vi "3D_plot.vi"(0 "Object Refnum In":refnum<vi>, 5 "error in (no error)":errorcluster, 7 "X":u16, 9 "Y":u16, 11 "Z":u16) -> (4 "3D Picture Control":refnum<vi>(3d-picture))   [LabVIEW 2012]
uses:
  <vilib>/Utility/miscctls.llb/LV3DPointTypeDef.ctl
  <vilib>/picture/3D Picture Control/NI_3D Picture Control.lvlib
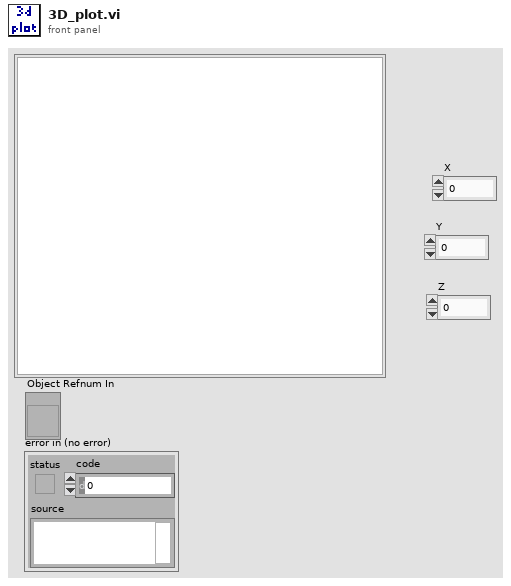
[diagram p1: front panel]
types:
  T1 = typedef "LV3DPointTypeDef.ctl" = cluster{"X":sgl, "Y":sgl, "Z":sgl}
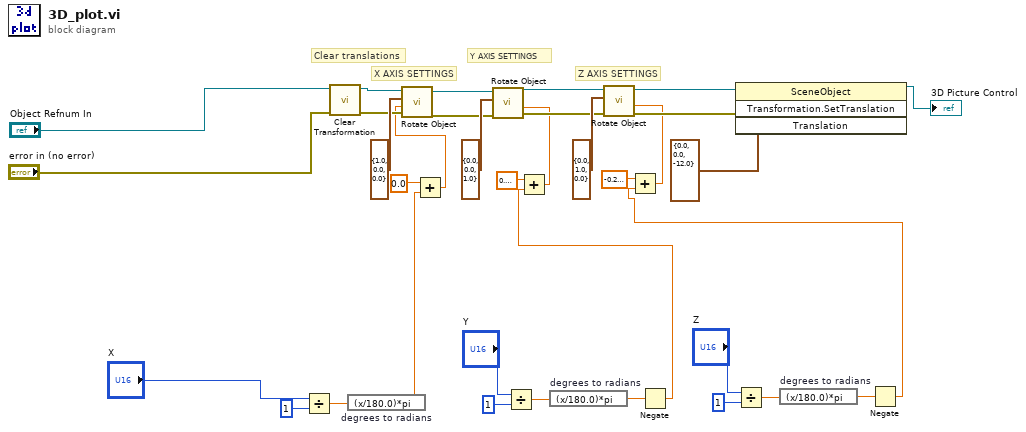
[diagram p0: block diagram]
diagram:
  # "Z AXIS SETTINGS"
  # "Y AXIS SETTINGS"
  # "Clear translations"
  # "X AXIS SETTINGS"
  n1 = Divide(x="X", y=1) -> (x/y=w15:dbl)
  n2 = call <vilib>:"Clear Transformation.vi"("error in (no error)"="error in (no error)", "Object Refnum In"="Object Refnum In") -> ("error out"=w24:errorcluster, "Object Refnum Out"=w34:refnum<vi>)  [unwired: 8 out]
  n3 = expression code="(x/180.0)*pi" "degrees to radians"(w15) -> (w14:dbl)
  n4 = Add(x=sgl 0.0 ("default X"), y=w14) -> (x+y=w22:dbl)
  n5 = call <vilib>:"Rotate Object.vi"("error in (no error)"=w24, "Angle"=w22, "Axis"=cluster{"X":sgl, "Y":sgl, "Z":sgl} {"X"=1.0, "Y"=0.0, "Z"=0.0}, "Scene.Object In"=w34) -> ("error out"=w25:errorcluster, "Scene.Object Out"=w26:refnum<vi>)  [unwired: 6 out]
  n6 = Divide(x="Y", y=1) -> (x/y=w12:dbl)
  n7 = expression code="(x/180.0)*pi" "degrees to radians"(w12) -> (w11:dbl)
  n8 = Negate(x=w11) -> (-x=w10:dbl)
  n9 = Add(x=sgl 0.6 ("default Y"), y=w10) -> (x+y=w19:dbl)
  n10 = call <vilib>:"Rotate Object.vi"("error in (no error)"=w25, "Angle"=w19, "Axis"=cluster{"X":sgl, "Y":sgl, "Z":sgl} {"X"=0.0, "Y"=0.0, "Z"=1.0}, "Scene.Object In"=w26) -> ("error out"=w27:errorcluster, "Scene.Object Out"=w28:refnum<vi>)  [unwired: 6 out]
  n11 = Divide(x="Z", y=1) -> (x/y=w4:dbl)
  n12 = expression code="(x/180.0)*pi" "degrees to radians"(w4) -> (w3:dbl)
  n13 = Negate(x=w3) -> (-x=w1:dbl)
  n14 = Add(x=sgl -0.2 ("Z"), y=w1) -> (x+y=w17:dbl)
  n15 = call <vilib>:"Rotate Object.vi"("error in (no error)"=w27, "Angle"=w17, "Axis"=cluster{"X":sgl, "Y":sgl, "Z":sgl} {"X"=0.0, "Y"=1.0, "Z"=0.0}, "Scene.Object In"=w28) -> ("error out"=w29:errorcluster, "Scene.Object Out"=w30:refnum<vi>)  [unwired: 6 out]
  n16 = invoke class="SceneObject" method="Transformation.SetTranslation"(reference=w30, error in=w29, "Translation"=T1 {"X"=0.0, "Y"=0.0, "Z"=-12.0}) -> (reference out=→"3D Picture Control":refnum<vi>)  [unwired: 1 in, 3 out]
